vi "Draw Picture based on Origin.vi"(6 "Not 32x32?":bool, 9 "Origin":T1, 11 "LayerIcon in":picture) -> (3 "LayerIcon out":picture)   [LabVIEW 2020, in "LabVIEW Icon API.lvlib"]
doc: "Apply the Origin information on the Picture."
uses:
  LabVIEW Icon API.lvlib
  <vilib>/Utility/miscctls.llb/LVPoint32TypeDef.ctl
  resource/plugins/lv_icon.lvlib
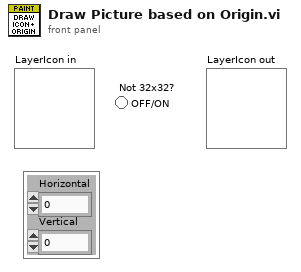
[diagram p1: front panel]
types:
  T1 = typedef "LVPoint32TypeDef.ctl" = cluster{"Horizontal":i32, "Vertical":i32}
  T2 = cluster{"left":i16, "top":i16, "right":i16, "bottom":i16}
  T3 = typedef "imagedata.ctl" = cluster{"image type":i32, "image depth":i32, "image":u8[], "mask":u8[], "colors":u32[], "Rectangle":cluster{"left":i16, "top":i16, "right":i16, "bottom":i16}}
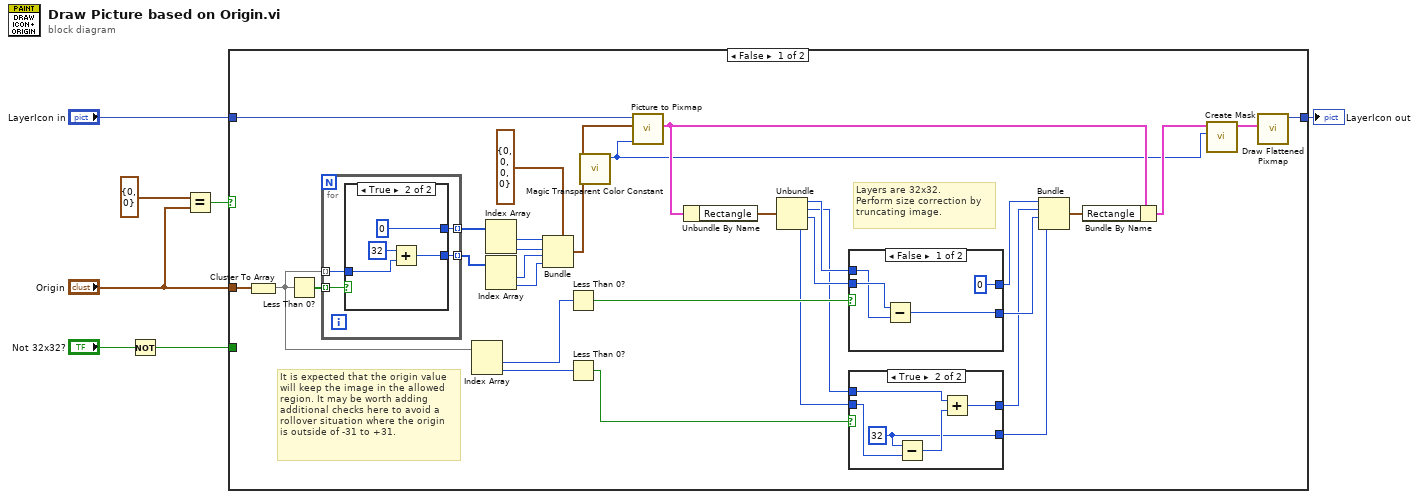
[diagram p0: block diagram]
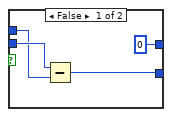
[diagram p2: hidden frame]
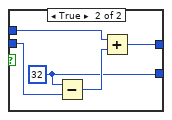
[diagram p3: hidden frame]
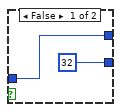
[diagram p4: hidden frame]
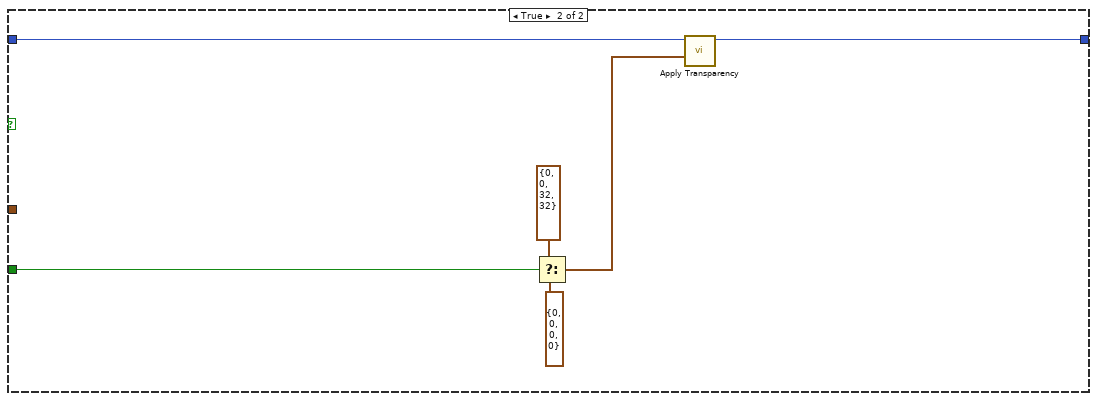
[diagram p5: hidden frame]
diagram:
  n1 = Not(x="Not 32x32?") -> (.not. x?=w5:bool)
  n2 = Equal?(x=T1 {"Horizontal"=0, "Vertical"=0} ("Origin"), y="Origin") -> (x = y?=w2:bool)
  n3 = case shown="False" w2 {
    tunnel: "LayerIcon in" -> [w38 w69]
    tunnel: "Origin" -> [w37 _]
    tunnel: [w27 w68] -> w1
    tunnel: w5 -> [_ w72]
    frame False {
      # "Layers are 32x32.\nPerform size correction by\ntruncating image."
      # "It is expected that the origin value\nwill keep the image in the allowed\nregion. It may be worth adding \nadditional checks here to avoid a\nrollover situation where the origin\nis outside of -31 to +31."
      n4 = Cluster To Array(cluster=w37) -> (array=w22:i32[])
      n5 = Less Than 0?(x=w22) -> (x < 0?=w36:bool[])
      n6 = for {
        tunnel: w36 -> [w60] mode=indexing
        tunnel: w22 -> [w59] mode=indexing
        tunnel: [w58] -> w35 mode=indexing
        tunnel: [w57] -> w34 mode=indexing
        n7 = case shown="True" w60 {
          tunnel: w59 -> [w61 w64]
          tunnel: [w61 0] -> w58
          tunnel: [32 w63] -> w57
          frame False {
          }
          frame True {
            n8 = Add(x=32, y=w64) -> (x+y=w63:i32)
          }
        }
      }
      n9 = Index Array(array=w22) -> (element #1=w21:i32, element #2=w12:i32)  [unwired: 2 in]
      n10 = Index Array(array=w35) -> (element #1=w31:i32, element #2=w30:i32)  [unwired: 2 in]
      n11 = Index Array(array=w34) -> (element #1=w29:i32, element #2=w28:i32)  [unwired: 2 in]
      n12 = Bundle(cluster=T2 {"left"=0, "top"=0, "right"=0, "bottom"=0} ("rect"), "left"=w31, "top"=w30, "right"=w29, "bottom"=w28) -> (w32:T2)
      n13 = Less Than 0?(x=w21) -> (x < 0?=w20:bool)
      n14 = Less Than 0?(x=w12) -> (x < 0?=w11:bool)
      n15 = call "Magic Transparent Color Constant.vi"() -> ("Magic transparent color constant"=w8:u32)  [unwired: 11 out]
      n16 = call <vilib>:"Picture to Pixmap.vi"("Background Color"=w8, "rect"=w32, "picture"=w38) -> ("image data"=w24:T3)  [unwired: 1 in, 7 out]
      n17 = Unbundle By Name(w24) -> ("Rectangle"=w23:T2)
      n18 = Unbundle(w23) -> ("left"=w19:i16, "top"=w14:i16, "right"=w18:i16, "bottom"=w13:i16)
      n19 = case shown="False" w20 {
        tunnel: w19 -> [w50 w54]
        tunnel: w18 -> [w51 w56]
        tunnel: [i16 0 w53] -> w17
        tunnel: [w49 w52] -> w16
        frame False {
          n20 = Subtract(x=w51, y=w50) -> (x-y=w49:i16)
        }
        frame True {
          w52 = i16 32 ("x")
          n21 = Subtract(x=w52, y=w56) -> (x-y=w55:i16)
          n22 = Add(x=w54, y=w55) -> (x+y=w53:i16)
        }
      }
      n23 = case shown="True" w11 {
        tunnel: w14 -> [w41 w45]
        tunnel: w13 -> [w42 w47]
        tunnel: [i16 0 w44] -> w10
        tunnel: [w40 w43] -> w9
        frame False {
          n24 = Subtract(x=w42, y=w41) -> (x-y=w40:i16)
        }
        frame True {
          w43 = i16 32 ("x")
          n25 = Subtract(x=w43, y=w47) -> (x-y=w46:i16)
          n26 = Add(x=w45, y=w46) -> (x+y=w44:i16)
        }
      }
      n27 = Bundle(w17, w10, "x"=w16, "x"=w9) -> (w15:cluster{i16, i16, "x":i16, "x":i16})  [unwired: 1 out]
      n28 = Bundle By Name(cluster=w24, "Rectangle"=w15) -> (w25:T3)
      n29 = call <vilib>:"Create Mask.vi"("Mask Color (Black)"=w8, "image data"=w25) -> ("image data"=w26:T3)  [unwired: 2 in, 7 out]
      n30 = call <vilib>:"Draw Flattened Pixmap.vi"("image data"=w26) -> ("new picture"=w27:picture)  [unwired: 1 in, 7 out]
    }
    frame True {
      n31 = Select(t=T2 {"left"=0, "top"=0, "right"=32, "bottom"=32} ("rect"), s=w72, f=T2 {"left"=0, "top"=0, "right"=0, "bottom"=0}) -> (s? t:f=w67:T2)
      n32 = call "Apply Transparency.vi"("rect"=w67, "in"=w69) -> ("out"=w68:picture)  [unwired: 9 out]
    }
  }
  "LayerIcon out" <- w1
